vi "Init.vi"(8 "error in (no error)":errorcluster, 11 "uService Template in":refnum<class "DAQ Manager.lvclass">) -> (0 "error out":errorcluster, 3 "uService Template out":refnum<class "DAQ Manager.lvclass">)   [LabVIEW 2020, in "DAQ Manager.lvlib" / "DAQ Manager.lvclass"]
uses:
  DAQ Manager.lvclass
  TALOS/TALOS_PPL.lvlibp/Interfaces/DAQ Control/DAQ Control.lvclass
  DAQ Manager.lvclass/DAQ Manager.ctl
  TALOS/TALOS_PPL.lvlibp
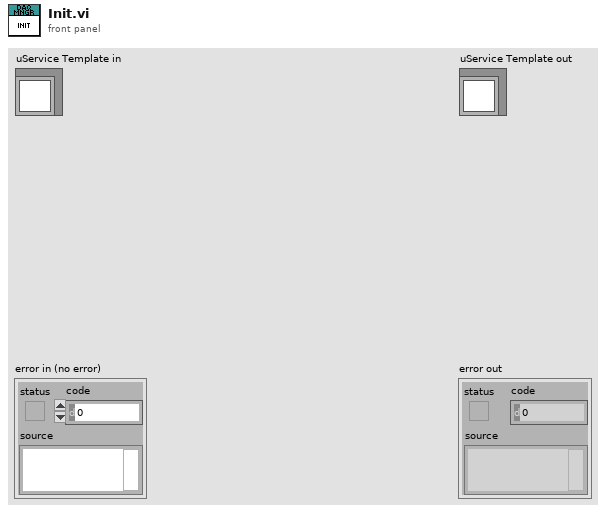
[diagram p1: front panel]
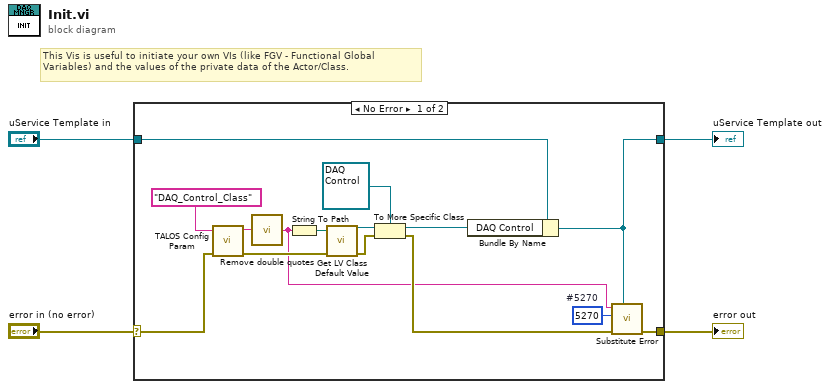
[diagram p0: block diagram]
diagram:
  # "This Vis is useful to initiate your own VIs (like FGV - Functional Global Variables) and the values of the private data of the Actor/Class."
  n1 = case shown="No Error" "error in (no error)" {
    selector: "error in (no error)" -> [w5 w20]
    tunnel: "uService Template in" -> [w18 w21]
    tunnel: [w10 w21] -> w4
    tunnel: [w8 w20] -> w3
    frame No Error {
      w13 = 5270  # #5270
      n2 = call "TALOS Config Param.vi"("error in (no error)"=w5, "Parameter Name"="DAQ_Control_Class") -> ("error out"=w19:errorcluster, "Output"=w6:string)  [unwired: 8 in]
      n3 = call "Remove double quotes.vi"("Input string"=w6) -> ("Output string"=w9:string)  [unwired: 4 in]
      n4 = String To Path(string=w9) -> (path=w17:path)
      n5 = call <vilib>:"Get LV Class Default Value.vi"("error in (no error)"=w19, "class path"=w17) -> ("error out"=w16:errorcluster, "object"=w15:refnum<class>)  [unwired: 8 in]
      n6 = To More Specific Class(target class=refnum<class "DAQ Control.lvclass"> refnum ("DAQ Control Interface"), reference=w15, error in=w16) -> (specific class reference=w11:refnum<class "DAQ Control.lvclass">, error out=w14:errorcluster)
      n7 = Bundle By Name(cluster=w18, "DAQ Control"=w11) -> (w10:refnum<class "DAQ Manager.lvclass">)
      n8 = call "Substitute Error.vi"("LabVIEW Object"=w10, "error in (no error)"=w14, "Error Code"=w13, "Optional String"=w9) -> ("error out"=w8:errorcluster)  [unwired: 7 in]
    }
    frame Error {
    }
  }
  "error out" <- w3
  "uService Template out" <- w4
